vi "Get XNET Signal Names.vi"(4 "Delete Olds?":bool, 6 "Add Info?":bool, 7 "Parent Ref in":T1 format="%.0x", 8 "error in":errorcluster, 9 "Tree In":refnum<vi>, 10 "Parent":string, 11 "Frms":refnum<k21>[](array[refnum])) -> (0 "error out":errorcluster, 1 "Tree Out":refnum<vi>, 3 "XNET Signal Names":refnum<k21>[](array[refnum]))   [LabVIEW 2023, in "Protection and Counter Addon System Explorer.lvlib"]
uses:
  Protection and Counter Addon System Explorer.lvlib
  <vilib>/NI VeriStand/Custom Device API/Custom Device Item Ref.ctl
  <vilib>/NI VeriStand/Custom Device API/Custom Device Channel.ctl
  <vilib>/NI VeriStand/Custom Device API/Custom Device Channel Type.ctl
  Addon Shared/SubVIs/GUID Lookup.vi
  <vilib>/NI VeriStand/Custom Device Tools/Custom Device Utility Library/NI VeriStand - Search for Item by Name.vi
  <vilib>/NI VeriStand/Custom Device API/Set Item Property (U32).vi
  <resource>/objmgr/xnet.rc
  <vilib>/NI VeriStand/Custom Device API/Custom Device API.lvlib
  Addon Shared/Protection and Counter Addon Shared.lvlib
  <vilib>/NI VeriStand/Custom Device Tools/Custom Device Utility Library/Custom Device Utility Library.lvlib
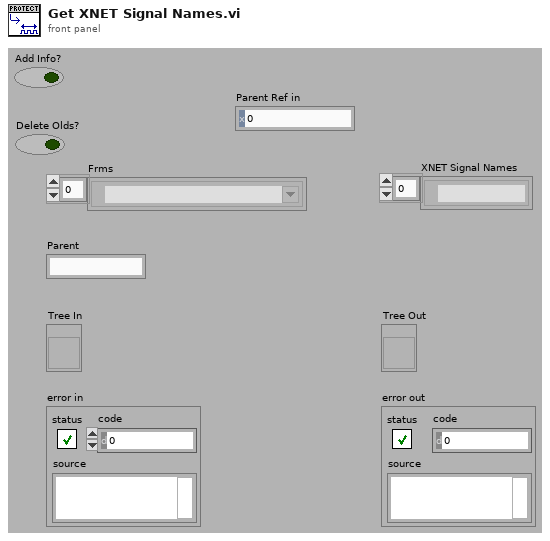
[diagram p1: front panel]
types:
  T1 = typedef "Custom Device API.lvlib/Custom Device Item Ref.ctl" = u64
  T2 = typedef "Custom Device API.lvlib/Custom Device Channel.ctl" = cluster{"Type":T3, "Units":string, "Default Value":dbl, "Faultable":bool, "Scalable":bool}
  T3 = typedef "Custom Device API.lvlib/Custom Device Channel Type.ctl" = enum16{"Input", "Output"}
  T4 = typedef "Custom Device API.lvlib/Custom Device Item Info.ctl" = cluster{"Name":string, "Is Channel":bool, "GUID":string, "Is Waveform":bool}
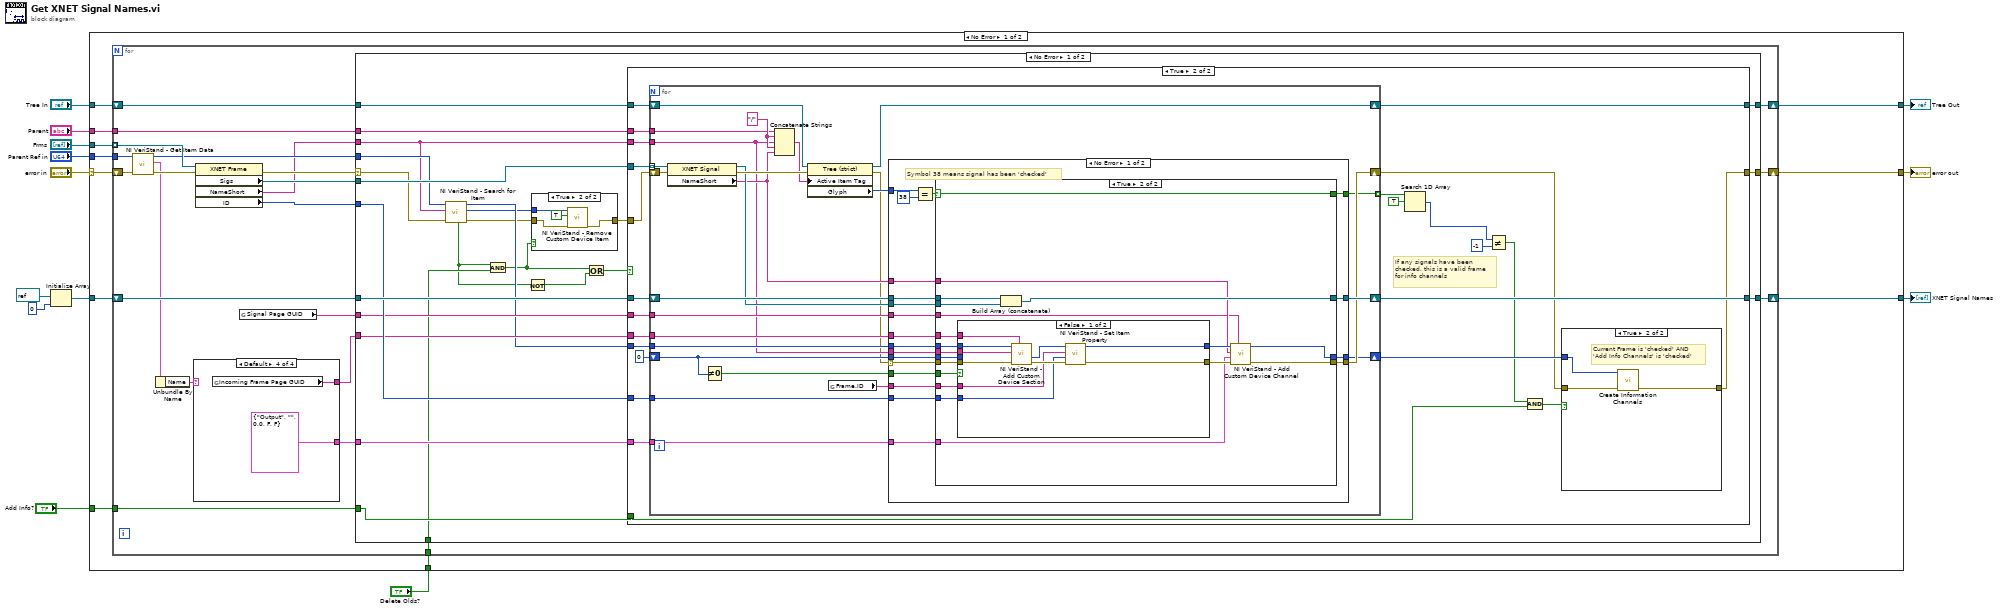
[diagram p0: block diagram]
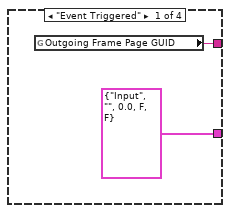
[diagram p2: hidden frame]
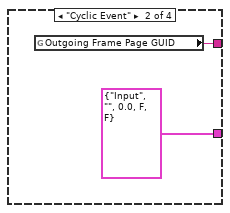
[diagram p3: hidden frame]
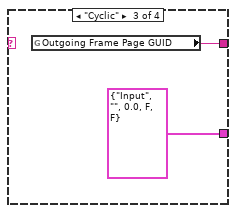
[diagram p4: hidden frame]
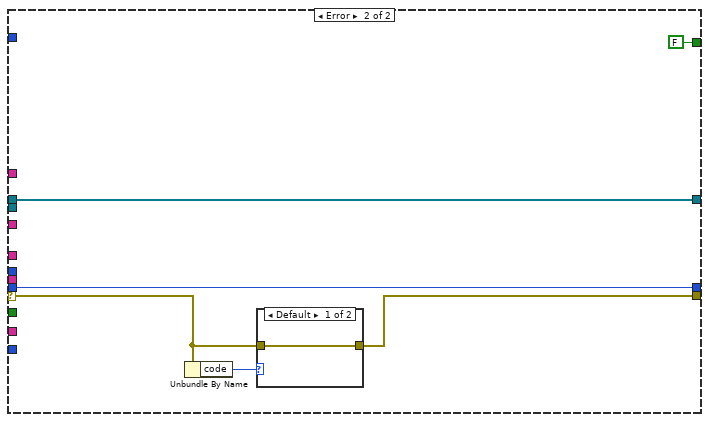
[diagram p9: hidden frame]
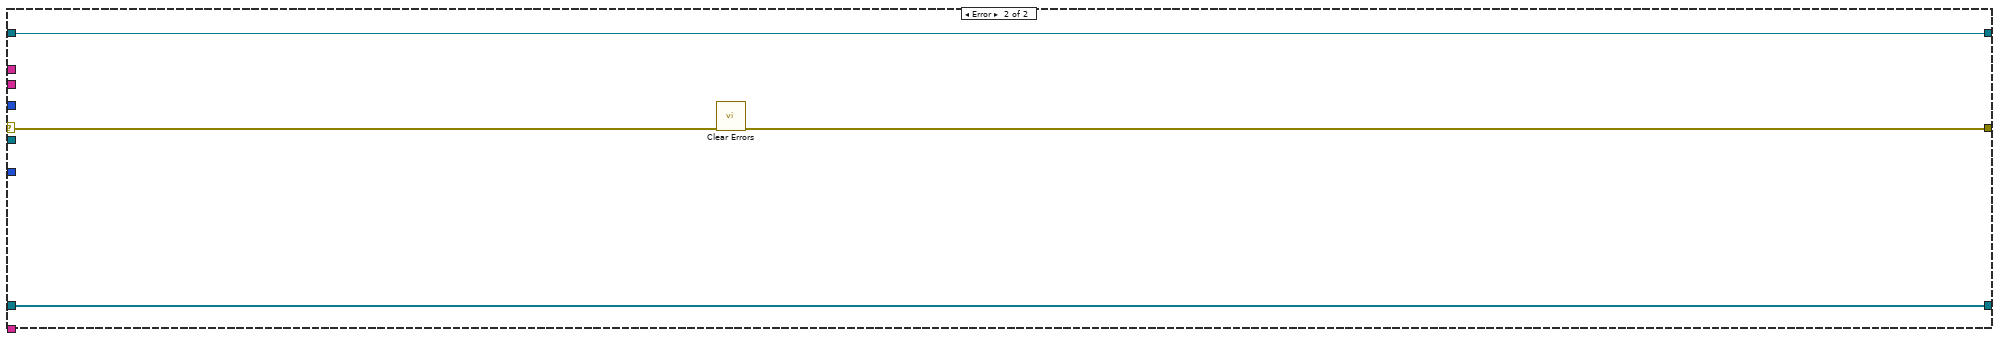
[diagram p12: hidden frame]
diagram:
  n1 = Initialize Array(refnum<k21> refnum ("XNET Signal"), 0 ("dimension size")) -> (w8:refnum<k21>[])
  n2 = case shown="No Error" "error in" {
    selector: "error in" -> [w21 w208]
    tunnel: "Parent" -> [w24 _]
    tunnel: [w23 w208] -> w3
    tunnel: "Frms" -> [w22 _]
    tunnel: [w20 _] -> w10
    tunnel: w8 -> [w19 _]
    tunnel: "Tree In" -> [w18 w207]
    tunnel: [w17 w207] -> w6
    tunnel: "Parent Ref in" -> [w16 _]
    tunnel: "Add Info?" -> [w15 _]
    tunnel: "Delete Olds?" -> [w14 _]
    frame No Error {
      n3 = for {
        shift-right: [w43] -> w23
        shift-left: w21 -> [w37]
        tunnel: w22 -> [w46] mode=indexing
        tunnel: w24 -> [w44]
        shift-right: [w40] -> w20
        shift-left: w19 -> [w41]
        shift-right: [w39] -> w17
        shift-left: w18 -> [w42]
        tunnel: w16 -> [w35]
        tunnel: w15 -> [w26]
        tunnel: w14 -> [w25]
        n4 = call <vilib>:"NI VeriStand - Get Item Data.vi"("error in (no error)"=w37, "Item Ref in"=w35) -> ("error out"=w36:errorcluster, "Item Info"=w33:T4, "Item Ref out"=w34:T1)  [unwired: 7 out]
        n5 = Unbundle By Name(w33) -> ("Name"=w32:string)
        n6 = case shown="Default" w32 {
          tunnel: [T2 {"Type"=enum."Input", "Units"="", "Default Value"=0.0, "Faultable"=FALSE, "Scalable"=FALSE} ("Channel") T2 {"Type"=enum."Input", "Units"="", "Default Value"=0.0, "Faultable"=FALSE, "Scalable"=FALSE} ("Channel") T2 {"Type"=enum."Input", "Units"="", "Default Value"=0.0, "Faultable"=FALSE, "Scalable"=FALSE} ("Channel") T2 {"Type"=enum."Output", "Units"="", "Default Value"=0.0, "Faultable"=FALSE, "Scalable"=FALSE} ("Channel")] -> w31
          tunnel: [w47 w49 w51 w53] -> w28
          frame "Event Triggered" {
            n7 = global read "GUID Lookup.vi" "Outgoing Frame Page GUID"() -> (w47:string)
          }
          frame "Cyclic Event" {
            n8 = global read "GUID Lookup.vi" "Outgoing Frame Page GUID"() -> (w49:string)
          }
          frame "Cyclic" {
            n9 = global read "GUID Lookup.vi" "Outgoing Frame Page GUID"() -> (w51:string)
          }
          frame Default {
            n10 = global read "GUID Lookup.vi" "Incoming Frame Page GUID"() -> (w53:string)
          }
        }
        n11 = property class="XNET Frame"(reference=w46, error in=w36) -> (error out=w38:errorcluster, "Sigs"=w45:refnum<k21>[], "NameShort"=w30:string, "ID"=w29:u32)  [unwired: 1 out]
        n12 = global read "GUID Lookup.vi" "Signal Page GUID"() -> (w27:string)
        n13 = case shown="No Error" w38 {
          selector: w38 -> [w70 w203]
          tunnel: w45 -> [w78 _]
          tunnel: w30 -> [w62 _]
          tunnel: w44 -> [w63 _]
          tunnel: [w64 w204] -> w43
          tunnel: w42 -> [w77 w205]
          tunnel: w41 -> [w76 w206]
          tunnel: [w75 w206] -> w40
          tunnel: [w61 w205] -> w39
          tunnel: w34 -> [w68 _]
          tunnel: w29 -> [w74 _]
          tunnel: w27 -> [w73 _]
          tunnel: w28 -> [w72 _]
          tunnel: w31 -> [w71 _]
          tunnel: w26 -> [w60 _]
          tunnel: w25 -> [w59 _]
          frame No Error {
            n14 = call-poly <vilib>:"NI VeriStand - Search for Item.vi"("error in"=w70, "Item Name"=w62, "Section Ref in"=w68) -> ("error out"=w66:errorcluster, "Item Ref"=w67:T1, "Section Ref out"=w69:T1, "Found"=w56:bool)  [unwired: 5 in]
            n15 = And(x=w56, y=w59) -> (x .and. y?=w58:bool)
            n16 = Not(x=w56) -> (.not. x?=w55:bool)
            n17 = case shown="True" w58 {
              tunnel: w67 -> [_ w202]
              tunnel: w66 -> [w198 w201]
              tunnel: [w198 w200] -> w65
              frame False {
              }
              frame True {
                n18 = call <vilib>:"NI VeriStand - Remove Custom Device Item.vi"("error in (no error)"=w201, "Force Delete (F)"=TRUE, "Item Ref in"=w202) -> ("error out"=w200:errorcluster)  [unwired: 7 in, 1 out]
              }
            }
            n19 = Or(x=w58, y=w55) -> (x .or. y?=w57:bool)
            n20 = case shown="True" w57 {
              tunnel: w78 -> [_ w105]
              tunnel: w77 -> [w81 w104]
              tunnel: w76 -> [w79 w103]
              tunnel: [w79 w102] -> w75
              tunnel: w74 -> [_ w100]
              tunnel: w73 -> [_ w99]
              tunnel: w72 -> [_ w98]
              tunnel: w71 -> [_ w97]
              tunnel: w69 -> [_ w96]
              tunnel: w65 -> [w80 w95]
              tunnel: [w80 w93] -> w64
              tunnel: w63 -> [_ w92]
              tunnel: w62 -> [_ w91]
              tunnel: [w81 w90] -> w61
              tunnel: w60 -> [_ w87]
              frame False {
              }
              frame True {
                # "If any signals have been\nchecked, this is a valid frame\nfor info channels"
                n21 = for {
                  tunnel: w105 -> [w135] mode=indexing
                  tunnel: w91 -> [w114]
                  tunnel: w92 -> [w132]
                  shift-right: [w124] -> w89
                  shift-left: w95 -> [w134]
                  shift-right: [w128] -> w102
                  shift-left: w103 -> [w127]
                  shift-right: [w125] -> w90
                  shift-left: w104 -> [w130]
                  tunnel: w96 -> [w123]
                  shift-right: [w122] -> w94
                  shift-left: T1 0 ("Parent Ref out") -> [w121]
                  tunnel: w100 -> [w118]
                  tunnel: w99 -> [w117]
                  tunnel: w98 -> [w116]
                  tunnel: w97 -> [w115]
                  tunnel: [w110] -> w84 mode=indexing
                  w133 = "/" ("string")
                  n22 = property class="XNET Signal"(reference=w135, error in=w134) -> (reference out=w126:refnum<k21>, error out=w131:errorcluster, "NameShort"=w119:string)
                  n23 = Not Equal To 0?(x=w121) -> (x != 0?=w120:bool)
                  n24 = Concatenate Strings(w132, w133, w114, w133, w119) -> (w111:string)
                  n25 = property class="Tree (strict)"(reference=w130, error in=w131, "Active Item Tag"=w111) -> (reference out=w125:refnum<vi>, error out=w113:errorcluster, "Glyph"=w129:i32)
                  n26 = global read "GUID Lookup.vi" "Frame.ID"() -> (w112:string)
                  n27 = case shown="No Error" w113 {
                    selector: w113 -> [w137 w193]
                    tunnel: w129 -> [w155 _]
                    tunnel: [w152 w195] -> w128
                    tunnel: w127 -> [w151 w195]
                    tunnel: w126 -> [w150 _]
                    tunnel: [w149 w192] -> w124
                    tunnel: w123 -> [w148 _]
                    tunnel: [w147 w196] -> w122
                    tunnel: w121 -> [w146 w196]
                    tunnel: w120 -> [w145 _]
                    tunnel: w119 -> [w144 _]
                    tunnel: w118 -> [w143 _]
                    tunnel: w112 -> [w142 _]
                    tunnel: w117 -> [w141 _]
                    tunnel: w116 -> [w140 _]
                    tunnel: w115 -> [w139 _]
                    tunnel: w114 -> [w138 _]
                    tunnel: [w136 FALSE] -> w110
                    frame No Error {
                      # "Symbol 38 means signal has been 'checked'"
                      n28 = Equal?(x=w155, y=38) -> (x = y?=w153:bool)
                      n29 = case shown="True" w153 {
                        selector: w153 -> [w156 w160]
                        tunnel: [w159 w176] -> w152
                        tunnel: w151 -> [w159 w178]
                        tunnel: w150 -> [_ w177]
                        tunnel: w145 -> [_ w175]
                        tunnel: w138 -> [_ w174]
                        tunnel: w137 -> [w158 w173]
                        tunnel: [w158 w161] -> w149
                        tunnel: w148 -> [_ w172]
                        tunnel: [w157 w169] -> w147
                        tunnel: w146 -> [w157 w171]
                        tunnel: w144 -> [_ w167]
                        tunnel: w140 -> [_ w166]
                        tunnel: w141 -> [_ w165]
                        tunnel: w143 -> [_ w164]
                        tunnel: w142 -> [_ w163]
                        tunnel: w139 -> [_ w162]
                        tunnel: [w156 w160] -> w136
                        frame False {
                        }
                        frame True {
                          n30 = case shown="False" w175 {
                            tunnel: w174 -> [w188 _]
                            tunnel: w173 -> [w187 w190]
                            tunnel: [w180 w190] -> w170
                            tunnel: w172 -> [w186 _]
                            tunnel: [w179 w189] -> w168
                            tunnel: w171 -> [_ w189]
                            tunnel: w166 -> [w185 _]
                            tunnel: w164 -> [w181 _]
                            tunnel: w163 -> [w182 _]
                            frame False {
                              n31 = call <vilib>:"NI VeriStand - Add Custom Device Section.vi"("GUID (Default Section)"=w185, "error in (no error)"=w187, "Section Name"=w188, "Parent Ref in"=w186) -> ("error out"=w183:errorcluster, "Section Ptr"=w184:T1)  [unwired: 4 in, 2 out]
                              n32 = call-poly <vilib>:"NI VeriStand - Set Item Property.vi"("error in (no error)"=w183, "Value"=w181, "Property Name"=w182, "Item Ref in"=w184) -> ("error out"=w180:errorcluster, "Item Ref out"=w179:T1)  [unwired: 5 in, 1 out]
                            }
                            frame True {
                            }
                          }
                          n33 = Build Array (concatenate)(w178, w177) -> (w176:refnum<k21>[])
                          n34 = call <vilib>:"NI VeriStand - Add Custom Device Channel.vi"("GUID (Default Channel)"=w165, "error in (no error)"=w170, "Channel"=w162, "Channel Name"=w167, "Parent Ref in"=w168) -> ("error out"=w161:errorcluster, "Parent Ref out"=w169:T1)  [unwired: 3 in, 2 out]
                        }
                      }
                    }
                    frame Error {
                      n35 = Unbundle By Name(w193) -> ("code"=w194:i32)
                      n36 = case shown="Default" w194 {
                        tunnel: [w197 _] -> w192
                        tunnel: w193 -> [w197 _]
                        frame Default {
                        }
                        frame 1136 {
                        }
                      }
                    }
                  }
                }
                n37 = Search 1D Array(1D array=w84, element=TRUE) -> (index of element=w82:i32)  [unwired: 1 in]
                n38 = Not Equal?(x=w82, y=-1) -> (x != y?=w86:bool)
                n39 = Compound Arithmetic op=AND(w86, w87) -> (w88:bool)
                n40 = case shown="True" w88 {
                  tunnel: w94 -> [_ w109]
                  tunnel: w89 -> [w106 w108]
                  tunnel: [w106 w107] -> w93
                  frame False {
                  }
                  frame True {
                    # "Current Frame is 'checked' AND\n'Add Info Channels' is 'checked'"
                    n41 = call "Create Information Channels.vi"("error in (no error)"=w108, "Node Ptr"=w109) -> ("error out"=w107:errorcluster)  [unwired: 8 in]
                  }
                }
              }
            }
          }
          frame Error {
            n42 = call <vilib>:"Clear Errors.vi"("error in (no error)"=w203) -> ("error out"=w204:errorcluster)  [unwired: 5 in, 1 out]
          }
        }
      }
    }
    frame Error {
    }
  }
  "error out" <- w3
  "XNET Signal Names" <- w10
  "Tree Out" <- w6
